vi "cmdJsonParse.vi"(8 "error in":errorcluster, 10 "controlStates":T1, 11 "cmdJson":string) -> (0 "error out":errorcluster, 2 "controlStates":T1, 3 "cmd":bool)   [LabVIEW 2024]
uses:
  Control/wsControlStates.ctl
  73fc7e1b-7bb7-4fdb-a00d-b5ca56efc9e0.vi
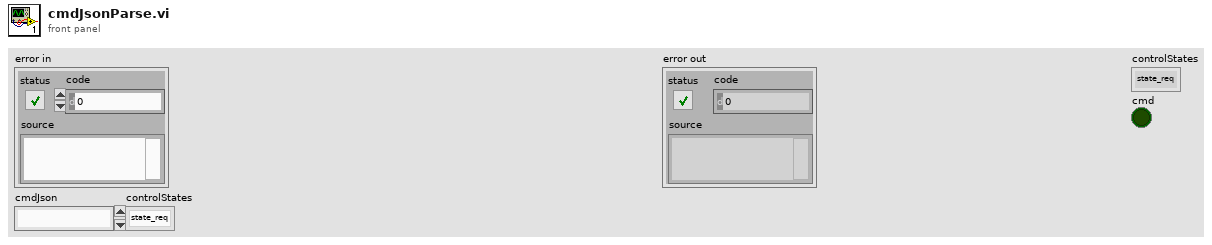
[diagram p1: front panel]
types:
  T1 = typedef "wsControlStates.ctl" = enum16{"state_req", "state_update", "entrySequence", "control", "exitSequence"}
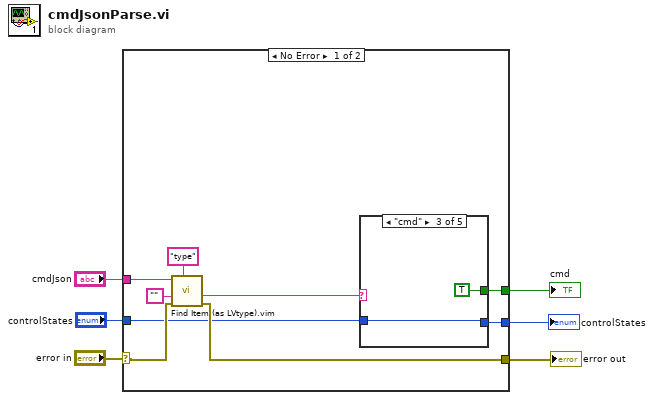
[diagram p0: block diagram]
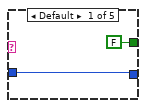
[diagram p2: hidden frame]
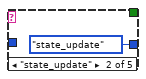
[diagram p3: hidden frame]
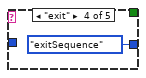
[diagram p4: hidden frame]
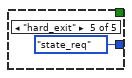
[diagram p5: hidden frame]
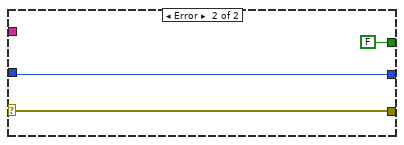
[diagram p6: hidden frame]
diagram:
  n1 = case shown="No Error" "error in" {
    selector: "error in" -> [w11 w25]
    tunnel: [w10 w25] -> w5
    tunnel: "controlStates" -> [w8 w23]
    tunnel: [w14 w23] -> w3
    tunnel: "cmdJson" -> [w13 _]
    tunnel: [w7 FALSE] -> w1
    frame No Error {
      n2 = call "Find Item (as LVtype).vim"("$Path or Item Name"="type", "error in (no error)"=w11, "Data Type and Default Value"="", "JSON"=w13) -> ("error out"=w10:errorcluster, "Data"=w9:string)  [unwired: 4 in, 2 out]
      n3 = case shown="\"cmd\"" w9 {
        tunnel: [w17 wsControlStates."state_update" ("Enum") w20 wsControlStates."exitSequence" ("controlStates") wsControlStates."state_req" ("controlStates")] -> w14
        tunnel: w8 -> [w17 _ w20 _ _]
        tunnel: [FALSE _ TRUE _ _] -> w7
        frame Default {
        }
        frame "state_update" {
        }
        frame "cmd" {
        }
        frame "exit" {
        }
        frame "hard_exit" {
        }
      }
    }
    frame Error {
    }
  }
  "error out" <- w5
  "controlStates" <- w3
  "cmd" <- w1
